vi "rs3 get frame data2.vi"(8 "error in (no error)":errorcluster, 11 "frame in":u64) -> (0 "error out":errorcluster, 1 "error":u64, 2 "image pointer out":u64, 3 "Frame out":u64)   [LabVIEW 2018, in "libRealSense3.lvlib"]
doc: "With a FRAME handle as input, this will return a pointer to the actual image data. \nUse the different MEMCOPY VIs to copy the data into LabVIEW."
uses:
  libRealSense3.lvlib
  realsense2.dll
panel:
  # "RS3 Get Frame Data 2"
  # "(C) Intel Corp. 2017,  AGJ"
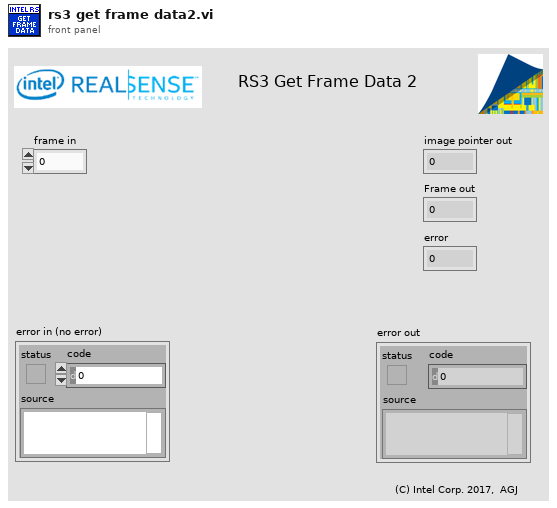
[diagram p1: front panel]
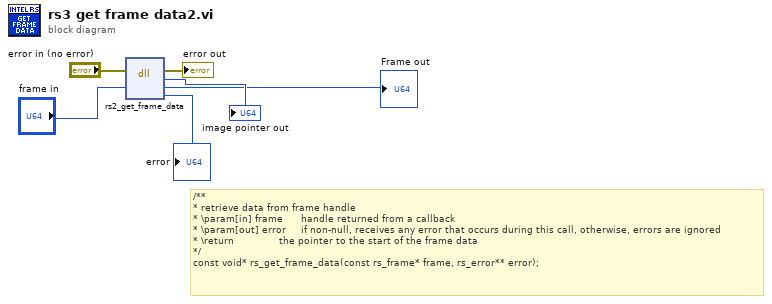
[diagram p0: block diagram]
diagram:
  # "/**\n* retrieve data from frame handle\n* \\param[in] frame      handle returned from a callback\n* \\param[out] error     if non-null, receives any error that occurs during this call, otherwise, errors are ignored\n* \\return               the pointer to the start of the frame data\n*/\nconst void* rs_get_frame_data(const rs_frame* frame, rs_error** error);"
  n1 = dll-call lib="C:/Users/aaron.jencks/Documents/Temp/realsense_labview_sdk/RealSense SDK2.11.0 for LabVIEW/realsense2.dll" fn="rs2_get_frame_data"(error in="error in (no error)", "frame"="frame in") -> (error out=→"error out":errorcluster, "return type"=→"image pointer out":u64, "frame"=→"Frame out":u64, "error"=→"error":u64)  [unwired: 3 in, 1 out]
